vi "LOERN_OnResize.vi"(0 "XRef":T10, 1 "Bounds":T8, 2 "Mouse Mods":T6, 3 "State In":T1={"Inputs"=1, "SelectedIndex"=1, "ClassInfo"=[]}) -> (14 "Reply":T4, 15 "Fatal Error Out":T3, 16 "State Out":T1={"Inputs"=1, "SelectedIndex"=1, "ClassInfo"=[]})   [LabVIEW 2016, in "LV Object Event Registration Node.xnode"]
uses:
  LV Object Event Registration Node.xnode
  <vilib>/XNodeSupport/XNodeXNodeRef.ctl
  <vilib>/XNodeSupport/XNodeRect32.ctl
  <vilib>/XNodeSupport/XNodeInt.ctl
  <vilib>/XNodeSupport/XNodeMouseMods.ctl
  <vilib>/XNodeSupport/XNodeBool.ctl
  LOERN_State.ctl
  LOERN_ClassInfo.ctl
  <vilib>/XNodeSupport/XNodeStringArray.ctl
  <vilib>/XNodeSupport/XNodeString.ctl
  <vilib>/XNodeSupport/XNodeErrorCluster.ctl
  <vilib>/XNodeSupport/NI_XNodeSupport.lvlib
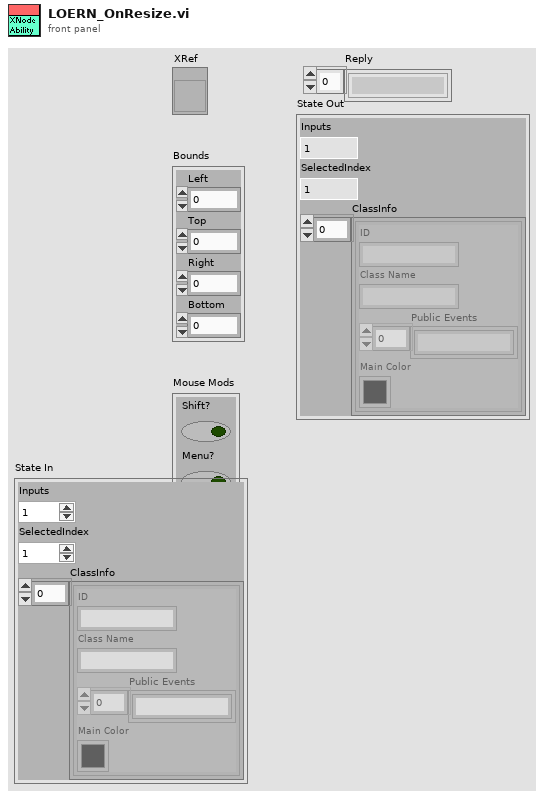
[diagram p1: front panel]
types:
  T1 = typedef "LV Object Event Registration Node.xnode/LOERN_State.ctl" = cluster{"Inputs":u16, "SelectedIndex":i16, "ClassInfo":T2[]}
  T2 = typedef "LV Object Event Registration Node.xnode/LOERN_ClassInfo.ctl" = cluster{"ID":string, "Class Name":string, "Public Events":string[], "Main Color":u32}
  T3 = typedef "NI_XNodeSupport.lvlib/XNodeErrorCluster.ctl" = errorcluster
  T4 = typedef "NI_XNodeSupport.lvlib/XNodeStringArray.ctl" = T5[]
  T5 = typedef "NI_XNodeSupport.lvlib/XNodeString.ctl" = string
  T6 = typedef "NI_XNodeSupport.lvlib/XNodeMouseMods.ctl" = cluster{"Shift?":T7, "Menu?":T7, "Alt?":T7}
  T7 = typedef "NI_XNodeSupport.lvlib/XNodeBool.ctl" = bool
  T8 = typedef "NI_XNodeSupport.lvlib/XNodeRect32.ctl" = cluster{"Left":T9, "Top":T9, "Right":T9, "Bottom":T9}
  T9 = typedef "NI_XNodeSupport.lvlib/XNodeInt.ctl" = i32
  T10 = typedef "NI_XNodeSupport.lvlib/XNodeXNodeRef.ctl" = refnum<vi>
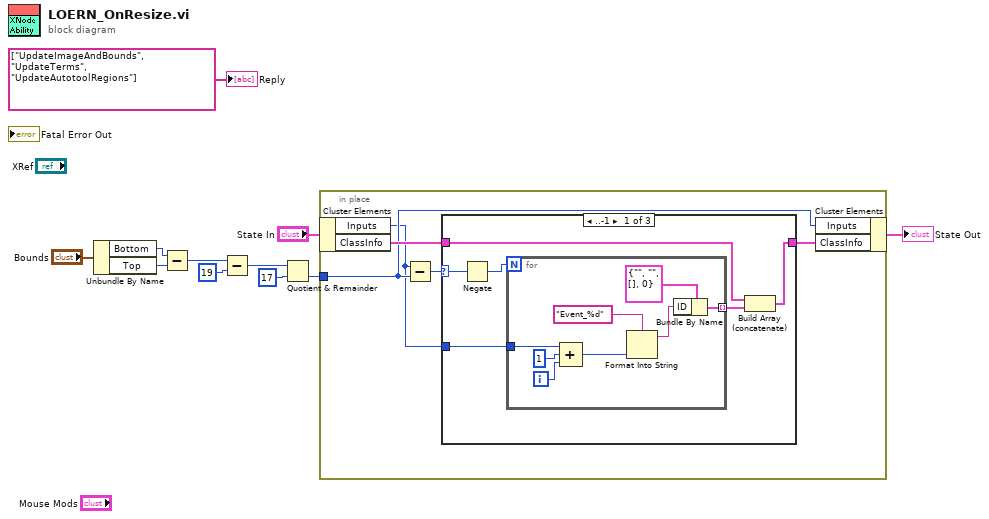
[diagram p0: block diagram]
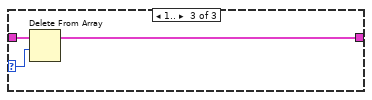
[diagram p3: hidden frame]
diagram:
  n1 = Unbundle By Name("Bounds") -> ("Bottom"=w9:T9, "Top"=w8:T9)
  n2 = Subtract(x=w9, y=w8) -> (x-y=w7:T9)
  n3 = Subtract(x=w7, y=19) -> (x-y=w5:T9)
  n4 = Quotient & Remainder(x=w5, y=17) -> (floor(x/y)=w2:T9)  [unwired: 1 out]
  n5 = in-place {
    in-place-border: w2 -> [w13]
    n6 = in-place-cluster #1("State In") -> ("Inputs"=w12:u16, "ClassInfo"=w15:T2[])
    n7 = Subtract(x=w12, y=w13) -> (x-y=w16:T9)
    n8 = case shown="..-1" w16 {
      selector: w16 -> [w18 _ w33]
      tunnel: w15 -> [w22 w31 w34]
      tunnel: [w21 w31 w32] -> w14
      tunnel: w12 -> [w20 _ _]
      frame ..-1 {
        n9 = Negate(x=w18) -> (-x=w17:T9)
        n10 = for {
          N: w17 -> [_]
          tunnel: w20 -> [w28]
          tunnel: [w23] -> w19 mode=indexing
          i -> [w29]
          n11 = Compound Arithmetic op=ADD(w28, u16 1 ("value"), w29) -> (w25:i32)
          n12 = Format Into String(format string="Event_%d", w25) -> (resulting string=w24:string)  [unwired: 2 in, 1 out]
          n13 = Bundle By Name(cluster=T2 {"ID"="", "Class Name"="", "Public Events"=[], "Main Color"=0} ("Cluster"), "ID"=w24) -> (w23:T2)
        }
        n14 = Build Array (concatenate)(w22, w19) -> (w21:T2[])
      }
      frame 0, Default {
      }
      frame 1.. {
        n15 = Delete From Array(array=w34, length=w33) -> (array with subset deleted=w32:T2[])  [unwired: 1 in, 1 out]
      }
    }
    n16 = in-place-cluster #1("Inputs"=w13, "ClassInfo"=w14) -> (→"State Out":T1)
  }
  "Reply" <- T4 ["UpdateImageAndBounds", "UpdateTerms", "UpdateAutotoolRegions"] ("Reply")
